vi "MAIN_Robot_Master.vi"() -> ()   [LabVIEW 2019]
uses:
  Type_defs/ESTADOS_ROBOT_MASTER.ctl
  Type_defs/TAREAS_ROBOT.ctl
  Type_defs/REFERENCIAS_CONTROLES_INDICADORES.ctl
  SHARED TYPES/Acciones_UI.ctl
  Type_defs/COMANDOS_TAREA.ctl
  <vilib>/Utility/error.llb/Error Cluster From Error Code.vi
  <vilib>/ErrorRing/Error Ring.xnode
  SHARED VI'S/SHARED VI'S.lvlib
  SHARED TYPES/SHARED TYPES.lvlib
panel:
  in  "Tab Control":enum32{"Page 1", "Page 2"}(tab)
  in  "Configurar estación":bool
  out "LABVIEW MESSAGES":string
  out "DISPOSITIVO CONECTADO":string
  out "ARDUINO MESSAGES":string
  in  "MOVIMIENTO MANUAL":bool
  in  "MOVER ASICS":bool
  in  "LEER QR":bool
  in  "TEST ASICS":bool
  in  "INICIAR COM":bool
  in  "Exit":bool
  out "ESTADO ACTUAL FSM":T1
  # "SISTEMA DE POSICIONAMIENTO AUTOMÁTICO DE ASICS"
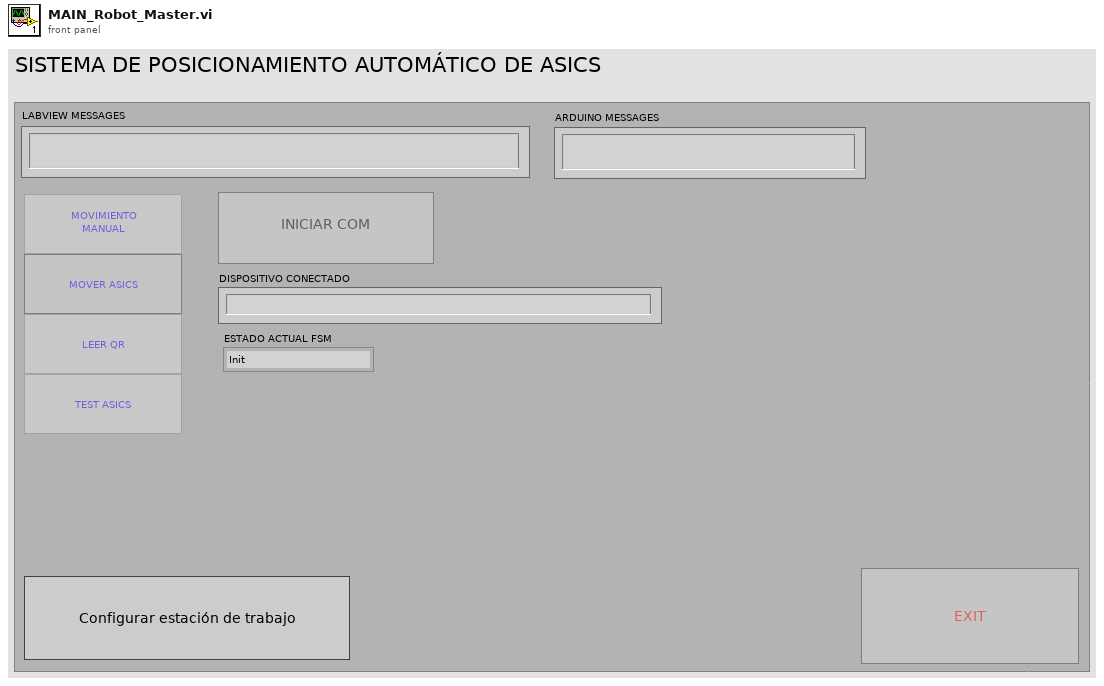
[diagram p1: front panel]
types:
  T1 = typedef "ESTADOS_ROBOT_MASTER.ctl" = enum16{"Init", "Iniciar Visa Arduino", "Sesiones Visa abiertas?", "Ping to Arduino", "Checkear config file", "Esperar_evento", "Tarea", "Exit", "Salir Arduino"}
  T2 = typedef "REFERENCIAS_CONTROLES_INDICADORES.ctl" = cluster{"LEER QR":refnum<vi>, "MOVER ASCIS":refnum<vi>, "CALIBRACION":refnum<vi>, "TEST ASICS":refnum<vi>, "EXIT":refnum<vi>, "AJUSTE CAM":refnum<vi>, "INICIAR COM":refnum<vi>, "ARDUINO MESSAGES":refnum<vi>, "LABVIEW MESSAGES":refnum<vi>, "DISPOSITIVO CONECTADO":refnum<vi>, "Config Estación":refnum<vi>}
  T3 = typedef "TAREAS_ROBOT.ctl" = enum16{"NINGUNA", "TEST ASICS", "AJUSTE CAM", "MOVER ASICS", "MOVIMIENTO MANUAL", "LEER QR", "CONFIG ESTACION"}
  T4 = typedef "SHARED TYPES.lvlib/Acciones_UI.ctl" = enum16{"Activar", "Desactivar", "Reiniciar default"}
  T5 = typedef "COMANDOS_TAREA.ctl" = enum16{"M", "T", "Q", "U", "S"}
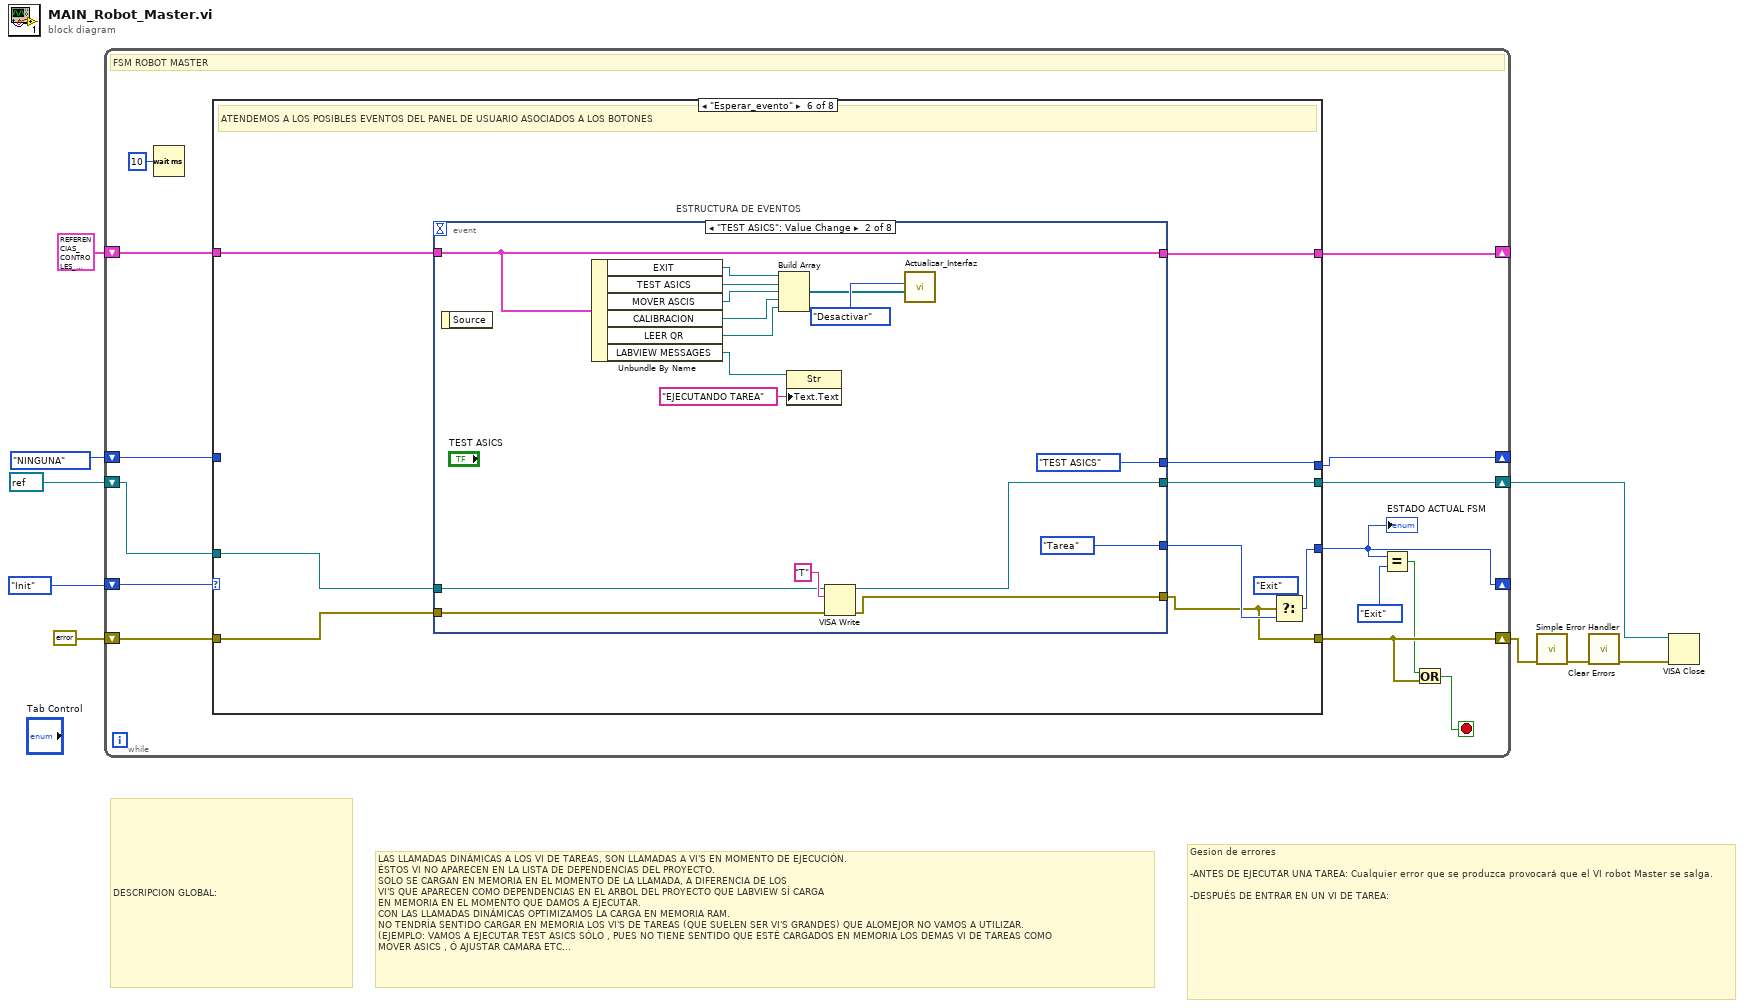
[diagram p0: block diagram]
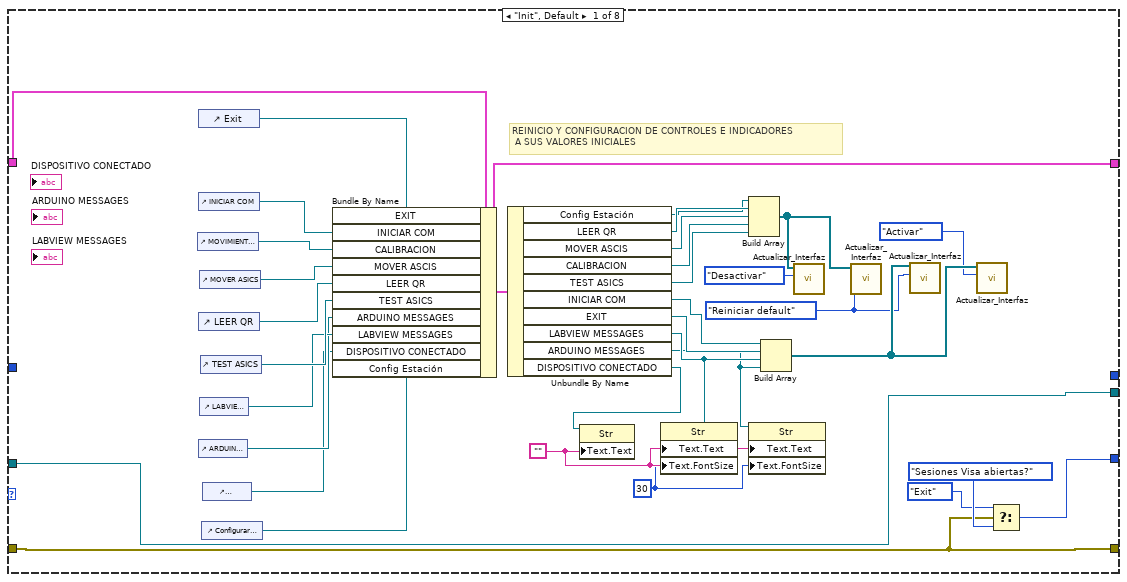
[diagram p2: hidden frame]
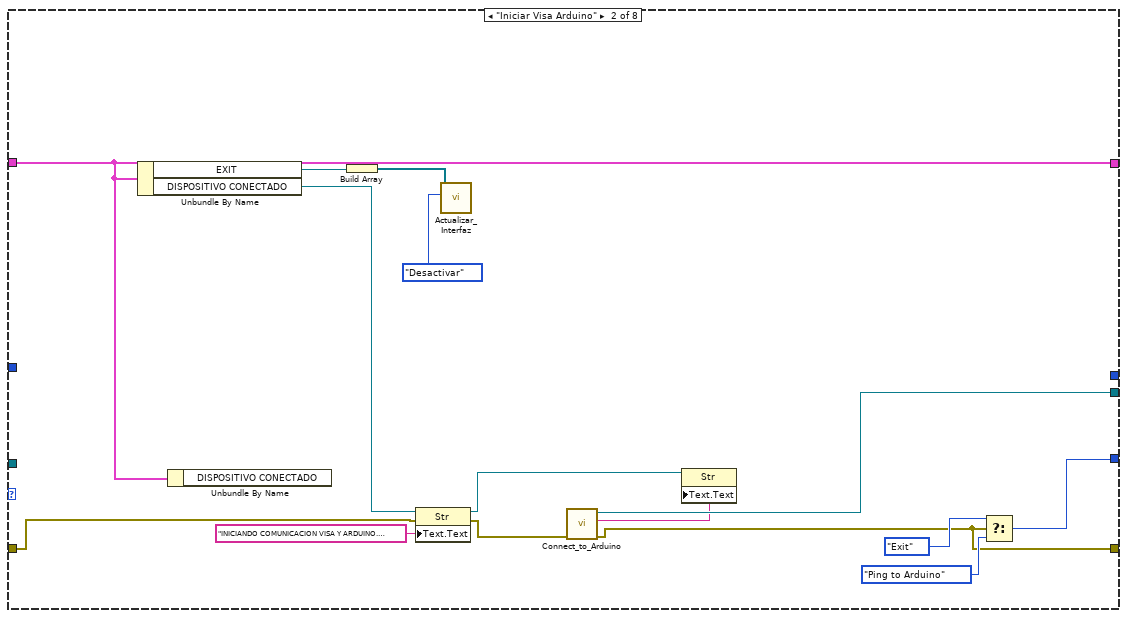
[diagram p3: hidden frame]
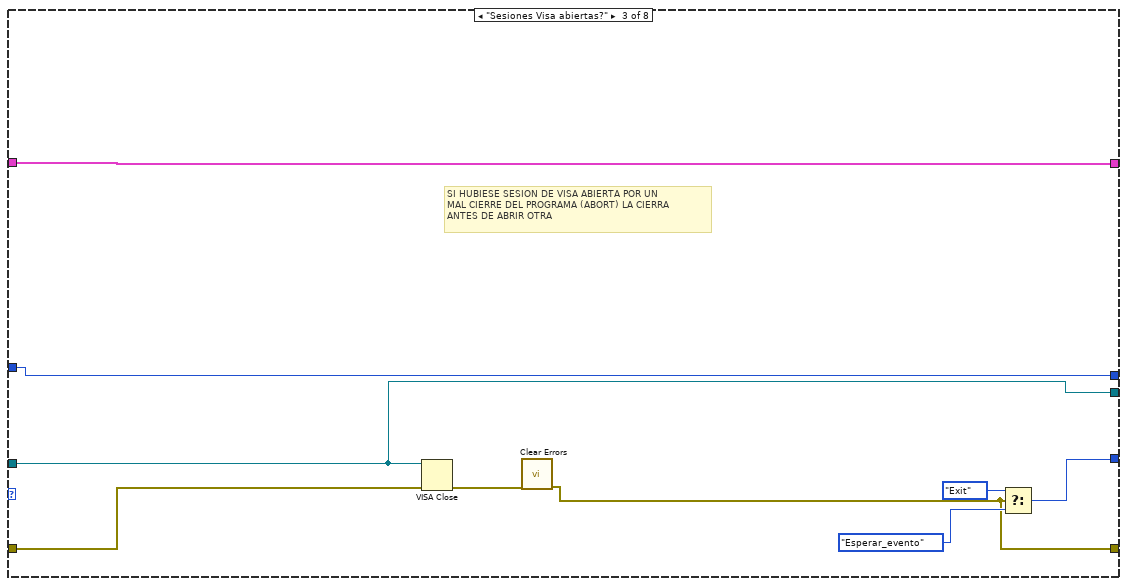
[diagram p4: hidden frame]
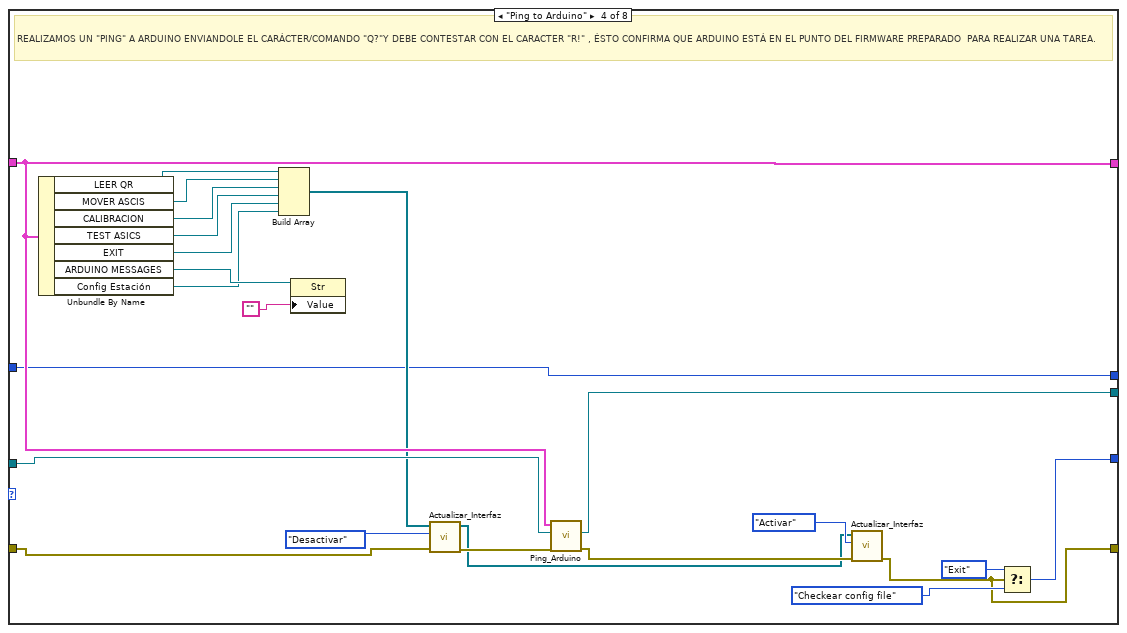
[diagram p5: hidden frame]
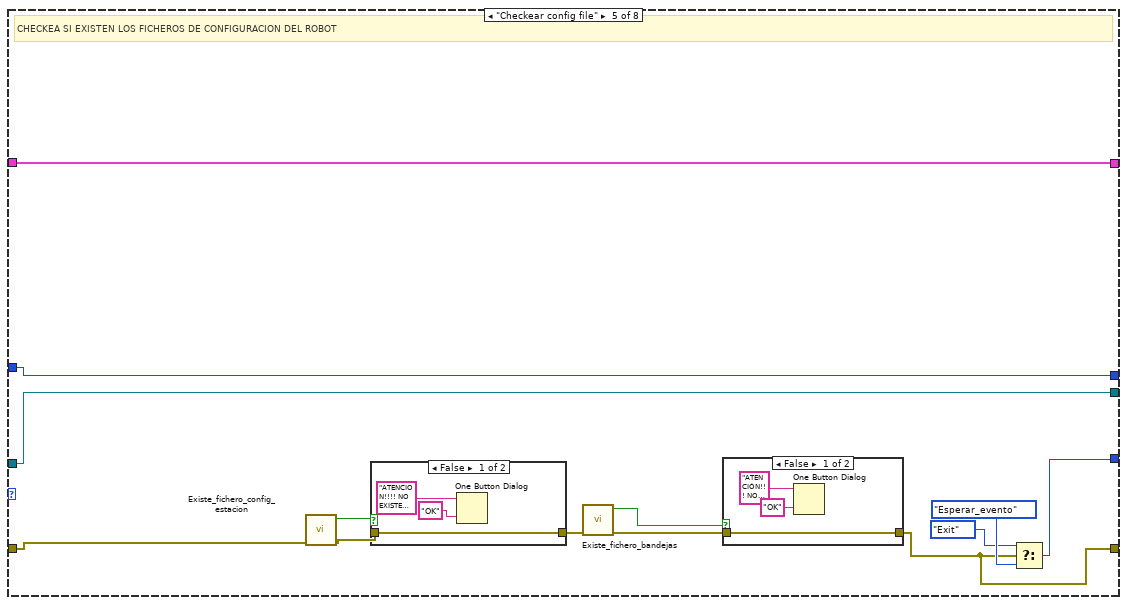
[diagram p6: hidden frame]
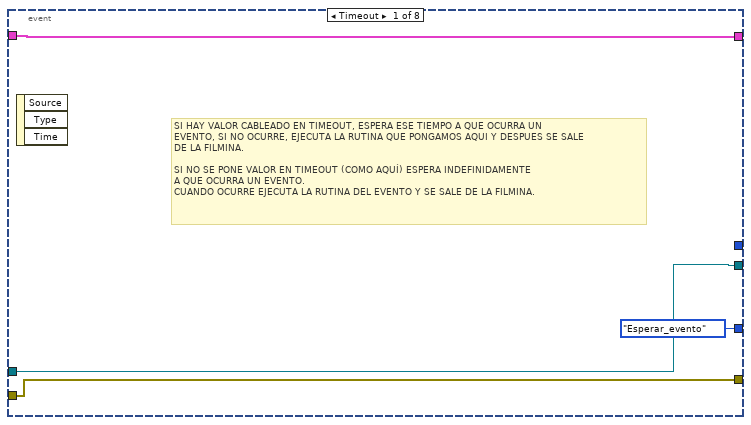
[diagram p9: hidden frame]
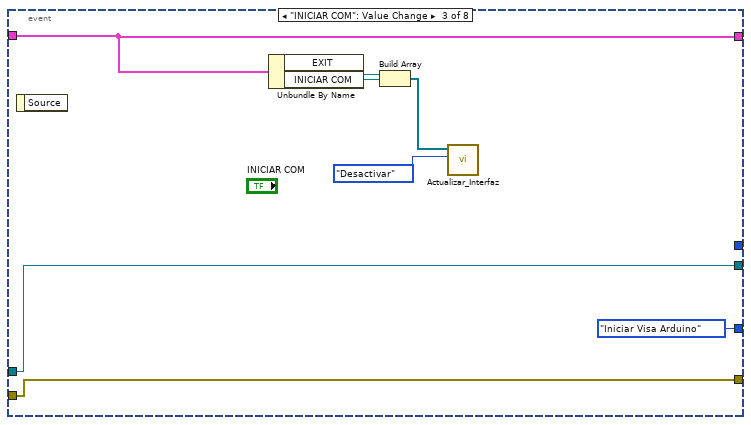
[diagram p10: hidden frame]
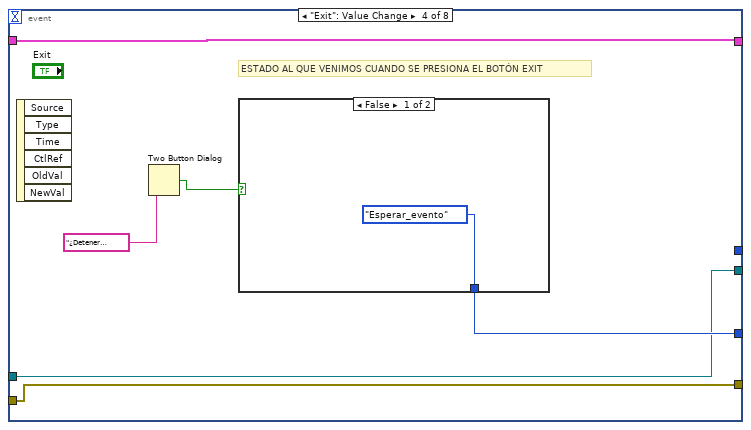
[diagram p11: hidden frame]
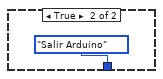
[diagram p12: hidden frame]
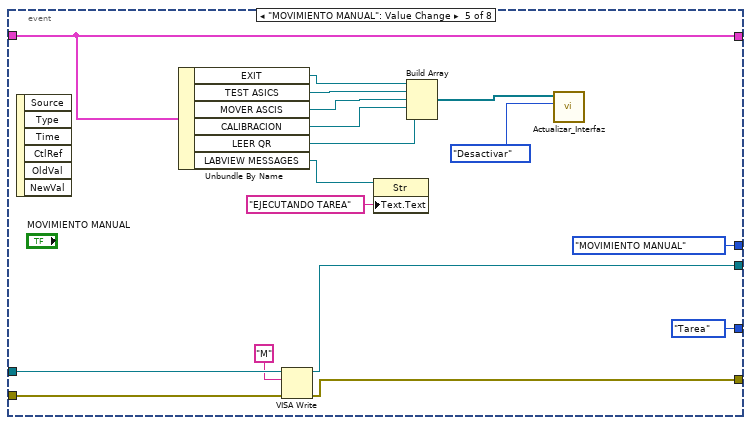
[diagram p13: hidden frame]
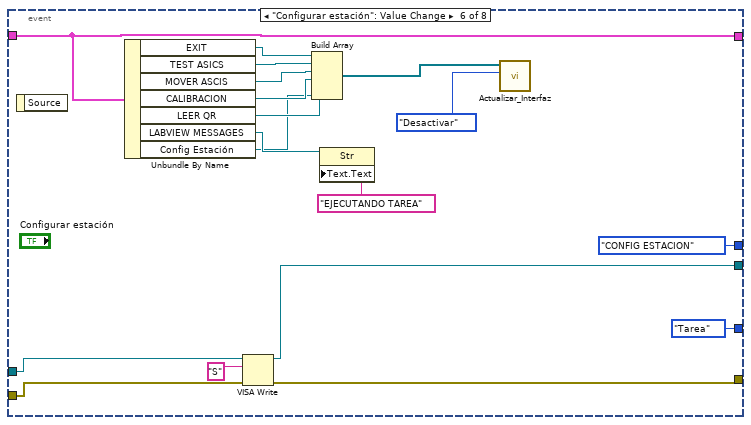
[diagram p14: hidden frame]
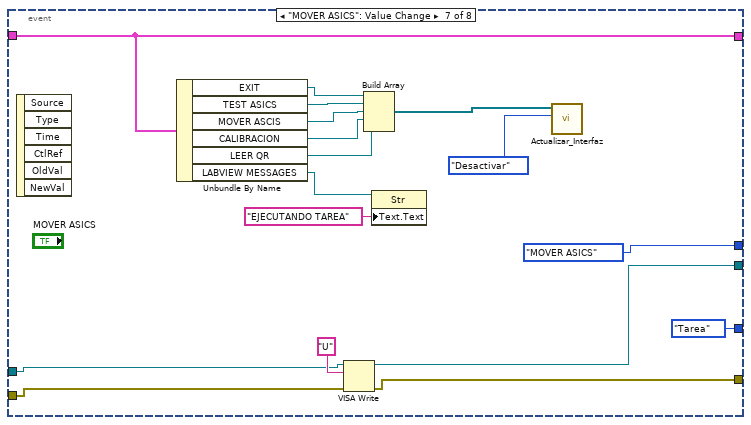
[diagram p15: hidden frame]
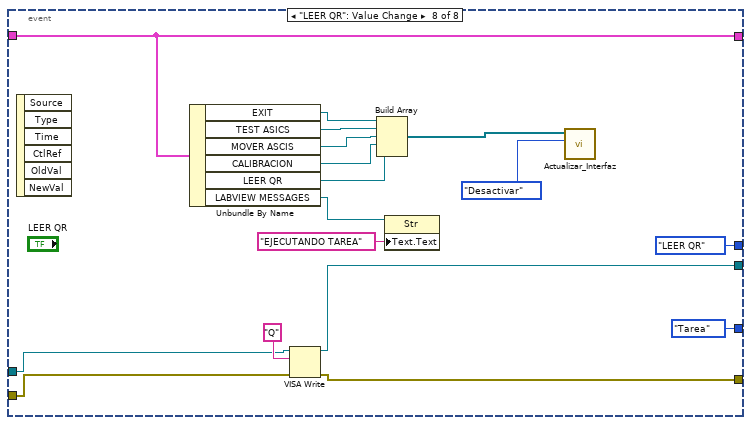
[diagram p16: hidden frame]
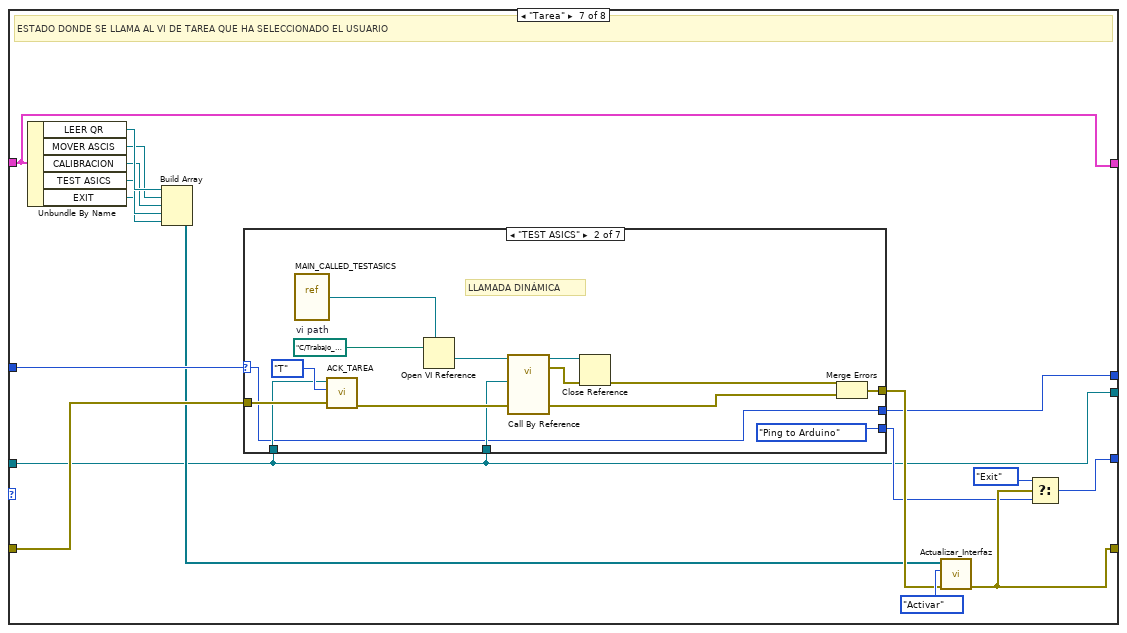
[diagram p17: hidden frame]
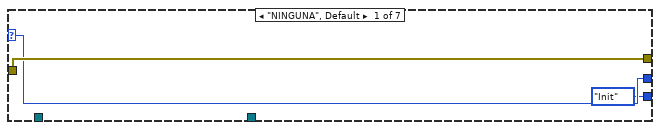
[diagram p18: hidden frame]
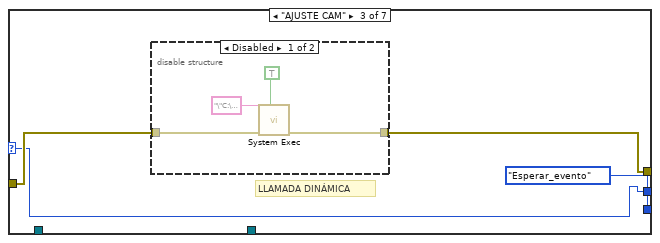
[diagram p19: hidden frame]
diagram:
  # "LAS LLAMADAS DINÁMICAS A LOS VI DE TAREAS, SON LLAMADAS A VI'S EN MOMENTO DE EJECUCIÓN.\nÉSTOS VI NO APARECEN EN LA LISTA DE DEPENDENCIAS DEL PROYECTO. \nSOLO SE CARGAN EN MEMORIA EN EL MOMENTO DE LA LLAMADA, A DIFERENCIA DE LOS\nVI'S QUE APARECEN COMO DEPENDENCIAS EN EL ARBOL DEL PROYECTO QUE LABVIEW SÍ CARGA\nEN MEMORIA EN EL MOMENTO QUE DAMOS A EJECUTAR.\nCON LAS LLAMADAS DINÁMICAS OPTIMIZAMOS LA CARGA EN MEMORIA RAM.\nNO TENDRÍA SENTIDO CARGAR EN MEMORIA LOS VI'S DE TAREAS (QUE SUELEN SER VI'S GRANDES) QUE ALOMEJOR NO VAMOS A UTILIZAR.\n(EJEMPLO: VAMOS A EJECUTAR TEST ASICS SÓLO , PUES NO TIENE SENTIDO QUE ESTÉ CARGADOS EN MEMORIA LOS DEMAS VI DE TAREAS COMO\nMOVER ASICS , Ó AJUSTAR CAMARA ETC..."
  # "Gesion de errores\n\n-ANTES DE EJECUTAR UNA TAREA: Cualquier error que se produzca provocará que el VI robot Master se salga.\n\n-DESPUÉS DE ENTRAR EN UN VI DE TAREA:"
  # "DESCRIPCION GLOBAL:"
  n1 = while {
    shift-right: [w15] -> _
    shift-left: ESTADOS_ROBOT_MASTER."Init" -> [w23]
    shift-right: [w18] -> w3
    shift-left: errorcluster {"status"=FALSE, "code"=0, "source"=""} ("error in (no error)") -> [w19]
    shift-right: [w20] -> _
    shift-left: T2 {"LEER QR"=refnum, "MOVER ASCIS"=refnum, "CALIBRACION"=refnum, "TEST ASICS"=refnum, "EXIT"=refnum, "AJUSTE CAM"=refnum, "INICIAR COM"=refnum, "ARDUINO MESSAGES"=refnum, "LABVIEW MESSAGES"=refnum, "DISPOSITIVO CONECTADO"=refnum, "Config Estación"=refnum} ("input cluster") -> [w21]
    shift-right: [w13] -> w2
    shift-left: refnum<visa-resource-name> refnum ("VISA resource name") -> [w10]
    shift-right: [w11] -> _
    shift-left: TAREAS_ROBOT."NINGUNA" -> [w12]
    stop <- w17 stop-if-true
    # "FSM ROBOT MASTER"
    n2 = Wait (ms)(milliseconds to wait=u32 10) -> ()  [unwired: 1 out]
    n3 = case shown="\"Esperar_evento\"" w23 {
      tunnel: w21 -> [w57 w67 w79 w102 w110 w135 w258 w359]
      tunnel: [w50 w67 w79 w102 w110 w134 w258 w359] -> w20
      tunnel: [w26 w58 w73 w85 w106 w127 w247 w355] -> w18
      tunnel: w19 -> [w26 w66 w81 w93 w117 w133 w245 w360]
      tunnel: [w27 w59 w74 w86 w105 w126 w248 ESTADOS_ROBOT_MASTER."Exit" ("Enum")] -> w15
      tunnel: w10 -> [w30 _ w78 w104 w109 w132 w243 w361]
      tunnel: [w30 w69 w78 w103 w109 w131 w243 w361] -> w13
      tunnel: w12 -> [_ _ w77 w89 w111 _ w250 w367]
      tunnel: [_ _ w77 w89 w111 w130 w242 w367] -> w11
      frame "Init", Default {
        w31 = 30
        w32 = ""
        w38 = Acciones_UI."Reiniciar default" ("Enum")
        # "REINICIO Y CONFIGURACION DE CONTROLES E INDICADORES\n A SUS VALORES INICIALES"
        n4 = control-ref of="MOVIMIENTO MANUAL"() -> (w54:refnum<vi>)
        n5 = control-ref of="Exit"() -> (w56:refnum<vi>)
        n6 = control-ref of="INICIAR COM"() -> (w55:refnum<vi>)
        n7 = control-ref of="LEER QR"() -> (w52:refnum<vi>)
        n8 = control-ref of="ARDUINO MESSAGES"() -> (w48:refnum<vi>)
        n9 = control-ref of="MOVER ASICS"() -> (w53:refnum<vi>)
        n10 = control-ref of="LABVIEW MESSAGES"() -> (w49:refnum<vi>)
        n11 = control-ref of="TEST ASICS"() -> (w51:refnum<vi>)
        n12 = control-ref of="Configurar estación"() -> (w25:refnum<vi>)
        n13 = control-ref of="DISPOSITIVO CONECTADO"() -> (w36:refnum<vi>)
        n14 = Bundle By Name(cluster=w57, "EXIT"=w56, "INICIAR COM"=w55, "CALIBRACION"=w54, "MOVER ASCIS"=w53, "LEER QR"=w52, "TEST ASICS"=w51, "ARDUINO MESSAGES"=w48, "LABVIEW MESSAGES"=w49, "DISPOSITIVO CONECTADO"=w36, "Config Estación"=w25) -> (w50:T2)
        n15 = Unbundle By Name(w50) -> ("Config Estación"=w24:refnum<vi>, "LEER QR"=w47:refnum<vi>, "MOVER ASCIS"=w46:refnum<vi>, "CALIBRACION"=w45:refnum<vi>, "TEST ASICS"=w44:refnum<vi>, "INICIAR COM"=w41:refnum<vi>, "EXIT"=w40:refnum<vi>, "LABVIEW MESSAGES"=w35:refnum<vi>, "ARDUINO MESSAGES"=w34:refnum<vi>, "DISPOSITIVO CONECTADO"=w33:refnum<vi>)
        n16 = property class="Str"(reference=w33, "Text.Text"=w32) -> ()  [unwired: 1 in, 2 out]
        n17 = property class="Str"(reference=w35, "Text.Text"=w32, "Text.FontSize"=w31) -> ()  [unwired: 1 in, 2 out]
        n18 = Build Array(w24, w47, w46, w45, w44) -> (w42:refnum<vi>[])
        n19 = property class="Str"(reference=w34, "Text.Text"=w32, "Text.FontSize"=w31) -> ()  [unwired: 1 in, 2 out]
        n20 = Build Array(w41, w40, w35, w34) -> (w39:refnum<vi>[])
        n21 = call "Actualizar_Interfaz.vi"("Enum"=Acciones_UI."Desactivar", "Controls"=w42) -> ()  [unwired: 8 in, 2 out]
        n22 = call "Actualizar_Interfaz.vi"("Enum"=w38, "Controls"=w42) -> ()  [unwired: 8 in, 2 out]
        n23 = call "Actualizar_Interfaz.vi"("Enum"=w38, "Controls"=w39) -> ()  [unwired: 8 in, 2 out]
        n24 = call "Actualizar_Interfaz.vi"("Enum"=Acciones_UI."Activar", "Controls"=w39) -> ()  [unwired: 8 in, 2 out]
        n25 = Select(t=ESTADOS_ROBOT_MASTER."Exit", s=w26, f=ESTADOS_ROBOT_MASTER."Sesiones Visa abiertas?" ("Enum")) -> (s? t:f=w27:T1)
      }
      frame "Iniciar Visa Arduino" {
        n26 = Unbundle By Name(w67) -> ("EXIT"=w72:refnum<vi>, "DISPOSITIVO CONECTADO"=w63:refnum<vi>)
        n27 = Unbundle By Name(w67) -> ()  [unwired: 1 out]
        n28 = Build Array(w72) -> (w71:refnum<vi>[])
        n29 = property class="Str"(reference=w63, error in=w66, "Text.Text"="INICIANDO COMUNICACION VISA Y ARDUINO. ESPERE...") -> (reference out=w62:refnum<vi>, error out=w64:errorcluster)
        n30 = call "Actualizar_Interfaz.vi"("Enum"=Acciones_UI."Desactivar", "Controls"=w71) -> ()  [unwired: 8 in, 2 out]
        n31 = call "Connect_to_Arduino.vi"("error in (no error)"=w64) -> ("error out"=w58:errorcluster, "DISPOSITIVO CONECTADO"=w68:string, "VISA Refnum out"=w69:refnum<visa-resource-name>)  [unwired: 8 in]
        n32 = property class="Str"(reference=w62, "Text.Text"=w68) -> ()  [unwired: 1 in, 2 out]
        n33 = Select(t=ESTADOS_ROBOT_MASTER."Exit", s=w58, f=ESTADOS_ROBOT_MASTER."Ping to Arduino" ("Enum")) -> (s? t:f=w59:T1)
      }
      frame "Sesiones Visa abiertas?" {
        # "SI HUBIESE SESION DE VISA ABIERTA POR UN \nMAL CIERRE DEL PROGRAMA (ABORT) LA CIERRA\nANTES DE ABRIR OTRA"
        n34 = VISA Close(VISA resource name=w78, error in (no error)=w81) -> (error out=w80:errorcluster)
        n35 = call <vilib>:"Clear Errors.vi"("error in (no error)"=w80) -> ("error out"=w73:errorcluster)  [unwired: 5 in, 1 out]
        n36 = Select(t=ESTADOS_ROBOT_MASTER."Exit", s=w73, f=ESTADOS_ROBOT_MASTER."Esperar_evento" ("Enum")) -> (s? t:f=w74:T1)
      }
      frame "Ping to Arduino" {
        # "REALIZAMOS UN \"PING\" A ARDUINO ENVIANDOLE EL CARÁCTER/COMANDO \"Q?\"Y DEBE CONTESTAR CON EL CARACTER \"R!\" , ÉSTO CONFIRMA QUE ARDUINO ESTÁ EN EL PUNTO DEL FIRMWARE PREPARADO  PARA REALIZAR UNA TAREA."
        n37 = Unbundle By Name(w102) -> ("LEER QR"=w101:refnum<vi>, "MOVER ASCIS"=w100:refnum<vi>, "CALIBRACION"=w99:refnum<vi>, "TEST ASICS"=w98:refnum<vi>, "EXIT"=w97:refnum<vi>, "ARDUINO MESSAGES"=w84:refnum<vi>, "Config Estación"=w82:refnum<vi>)
        n38 = Build Array(w101, w100, w99, w98, w97, w82) -> (w95:refnum<vi>[])
        n39 = property class="Str"(reference=w84, "Value"="") -> ()  [unwired: 1 in, 2 out]
        n40 = call "Actualizar_Interfaz.vi"("error in (no error)"=w93, "Enum"=Acciones_UI."Desactivar", "Controls"=w95) -> ("error out"=w94:errorcluster, "Controls 2"=w90:refnum<vi>[])  [unwired: 7 in]
        n41 = call "Ping_Arduino.vi"("error in (no error)"=w94, "VISA resource name"=w104, "input cluster"=w102) -> ("error IO"=w91:errorcluster, "VISA resource name out"=w103:refnum<visa-resource-name>)  [unwired: 7 in]
        n42 = call "Actualizar_Interfaz.vi"("error in (no error)"=w91, "Enum"=Acciones_UI."Activar", "Controls"=w90) -> ("error out"=w85:errorcluster)  [unwired: 7 in, 1 out]
        n43 = Select(t=ESTADOS_ROBOT_MASTER."Exit", s=w85, f=ESTADOS_ROBOT_MASTER."Checkear config file" ("Enum")) -> (s? t:f=w86:T1)
      }
      frame "Checkear config file" {
        # "CHECKEA SI EXISTEN LOS FICHEROS DE CONFIGURACION DEL ROBOT"
        n44 = call "Existe_fichero_config_estacion.vi"("Error In"=w117) -> ("Error Out"=w115:errorcluster, "file or folder exists?"=w116:bool)  [unwired: 9 in]
        n45 = case shown="False" w116 {
          tunnel: w115 -> [w122 w125]
          tunnel: [w122 w125] -> w114
          frame False {
            n46 = One Button Dialog(message="ATENCION!!!! NO EXISTE FICHERO DE CONFIGURACIÓN DE ESTACION\nEN EL DIRECTORIO RAÍZ DE ROBOT MASTER ", button name ("OK")="OK") -> ()  [unwired: 1 out]
          }
          frame True {
          }
        }
        n47 = call "Existe_fichero_bandejas.vi"("Error In"=w114) -> ("Error Out"=w112:errorcluster, "existe fichero bandejas?"=w113:bool)  [unwired: 9 in]
        n48 = case shown="False" w113 {
          tunnel: w112 -> [w118 w121]
          tunnel: [w118 w121] -> w106
          frame False {
            n49 = One Button Dialog(message="ATENCIÓN!!! NO EXISTE FICHERO DE CONFIGURACION DE BANDEJAS \".db\"\nEN EL DIRECTORIO RAIZ DE ROBOT MASTER.", button name ("OK")="OK") -> ()  [unwired: 1 out]
          }
          frame True {
          }
        }
        n50 = Select(t=ESTADOS_ROBOT_MASTER."Exit", s=w106, f=ESTADOS_ROBOT_MASTER."Esperar_evento" ("Enum")) -> (s? t:f=w105:T1)
      }
      frame "Esperar_evento" {
        # "ATENDEMOS A LOS POSIBLES EVENTOS DEL PANEL DE USUARIO ASOCIADOS A LOS BOTONES"
        n51 = event "ESTRUCTURA DE EVENTOS" shown="[1] \"TEST ASICS\": Value Change" {
          selector: _ -> [_ _ _ _ _ _ _ _]
          dyn-events: _ -> [_ _ _ _ _ _ _ _]
          timeout: _ -> [_ _ _ _ _ _ _ _]
          tunnel: w135 -> [w136 w147 w160 w165 w175 w192 w215 w232]
          tunnel: [ESTADOS_ROBOT_MASTER."Esperar_evento" ("Enum") ESTADOS_ROBOT_MASTER."Tarea" ("Enum") ESTADOS_ROBOT_MASTER."Iniciar Visa Arduino" ("Enum") w168 ESTADOS_ROBOT_MASTER."Tarea" ("Enum") ESTADOS_ROBOT_MASTER."Tarea" ("Enum") ESTADOS_ROBOT_MASTER."Tarea" ("Enum") ESTADOS_ROBOT_MASTER."Tarea" ("Enum")] -> w129
          tunnel: [w136 w147 w160 w165 w175 w192 w215 w232] -> w134
          tunnel: w133 -> [w139 w143 w157 w166 w178 w197 w212 w228]
          tunnel: [w139 w142 w157 w166 w176 w196 w209 w227] -> w127
          tunnel: w132 -> [w138 w141 w159 w167 w180 w198 w211 w226]
          tunnel: [w138 w140 w159 w167 w177 w195 w210 w225] -> w131
          tunnel: [_ TAREAS_ROBOT."TEST ASICS" _ _ TAREAS_ROBOT."MOVIMIENTO MANUAL" TAREAS_ROBOT."CONFIG ESTACION" TAREAS_ROBOT."MOVER ASICS" TAREAS_ROBOT."LEER QR"] -> w130
          event Timeout {
            # "SI HAY VALOR CABLEADO EN TIMEOUT, ESPERA ESE TIEMPO A QUE OCURRA UN \nEVENTO, SI NO OCURRE, EJECUTA LA RUTINA QUE PONGAMOS AQUI Y DESPUES SE SALE\nDE LA FILMINA.\n\nSI NO SE PONE VALOR EN TIMEOUT (COMO AQUÍ) ESPERA INDEFINIDAMENTE \nA QUE OCURRA UN EVENTO.\nCUANDO OCURRE EJECUTA LA RUTINA DEL EVENTO Y SE SALE DE LA FILMINA."
            n52 = event-data() -> ()  [unwired: 1 in, 3 out]
          }
          event "TEST ASICS": Value Change {
            n53 = event-data() -> ()  [unwired: 1 in, 1 out]
            n54 = Unbundle By Name(w147) -> ("EXIT"=w145:refnum<vi>, "TEST ASICS"=w154:refnum<vi>, "MOVER ASCIS"=w153:refnum<vi>, "CALIBRACION"=w152:refnum<vi>, "LEER QR"=w151:refnum<vi>, "LABVIEW MESSAGES"=w149:refnum<vi>)
            n55 = Build Array(w145, w154, w153, w152, w151) -> (w150:refnum<vi>[])
            n56 = property class="Str"(reference=w149, "Text.Text"="EJECUTANDO TAREA") -> ()  [unwired: 1 in, 2 out]
            n57 = VISA Write(VISA resource name=w141, write buffer="T", error in (no error)=w143) -> (VISA resource name out=w140:refnum<visa-resource-name>, error out=w142:errorcluster)  [unwired: 1 out]
            n58 = call "Actualizar_Interfaz.vi"("Enum"=Acciones_UI."Desactivar", "Controls"=w150) -> ()  [unwired: 8 in, 2 out]
          }
          event "INICIAR COM": Value Change {
            n59 = event-data() -> ()  [unwired: 1 in, 1 out]
            n60 = Unbundle By Name(w160) -> ("EXIT"=w163:refnum<vi>, "INICIAR COM"=w158:refnum<vi>)
            n61 = Build Array(w163, w158) -> (w162:refnum<vi>[])
            n62 = call "Actualizar_Interfaz.vi"("Enum"=Acciones_UI."Desactivar", "Controls"=w162) -> ()  [unwired: 8 in, 2 out]
          }
          event "Exit": Value Change {
            # "ESTADO AL QUE VENIMOS CUANDO SE PRESIONA EL BOTÓN EXIT"
            n63 = event-data() -> ()  [unwired: 1 in, 6 out]
            n64 = Two Button Dialog(message="¿Detener ejecución?") -> (T button?=w169:bool)  [unwired: 2 in]
            n65 = case shown="False" w169 {
              tunnel: [ESTADOS_ROBOT_MASTER."Esperar_evento" ("Enum") ESTADOS_ROBOT_MASTER."Salir Arduino" ("Enum")] -> w168
              frame False {
              }
              frame True {
              }
            }
          }
          event "MOVIMIENTO MANUAL": Value Change {
            n66 = event-data() -> ()  [unwired: 1 in, 6 out]
            n67 = Unbundle By Name(w175) -> ("EXIT"=w173:refnum<vi>, "TEST ASICS"=w188:refnum<vi>, "MOVER ASCIS"=w187:refnum<vi>, "CALIBRACION"=w186:refnum<vi>, "LEER QR"=w185:refnum<vi>, "LABVIEW MESSAGES"=w183:refnum<vi>)
            n68 = VISA Write(VISA resource name=w180, write buffer="M", error in (no error)=w178) -> (VISA resource name out=w177:refnum<visa-resource-name>, error out=w176:errorcluster)  [unwired: 1 out]
            n69 = property class="Str"(reference=w183, "Text.Text"="EJECUTANDO TAREA") -> ()  [unwired: 1 in, 2 out]
            n70 = Build Array(w173, w188, w187, w186, w185) -> (w184:refnum<vi>[])
            n71 = call "Actualizar_Interfaz.vi"("Enum"=Acciones_UI."Desactivar", "Controls"=w184) -> ()  [unwired: 8 in, 2 out]
          }
          event "Configurar estación": Value Change {
            n72 = event-data() -> ()  [unwired: 1 in, 1 out]
            n73 = Unbundle By Name(w192) -> ("EXIT"=w190:refnum<vi>, "TEST ASICS"=w206:refnum<vi>, "MOVER ASCIS"=w205:refnum<vi>, "CALIBRACION"=w204:refnum<vi>, "LEER QR"=w203:refnum<vi>, "LABVIEW MESSAGES"=w201:refnum<vi>, "Config Estación"=w191:refnum<vi>)
            n74 = VISA Write(VISA resource name=w198, write buffer="S", error in (no error)=w197) -> (VISA resource name out=w195:refnum<visa-resource-name>, error out=w196:errorcluster)  [unwired: 1 out]
            n75 = Build Array(w190, w206, w205, w204, w203, w191) -> (w202:refnum<vi>[])
            n76 = property class="Str"(reference=w201, "Text.Text"="EJECUTANDO TAREA") -> ()  [unwired: 1 in, 2 out]
            n77 = call "Actualizar_Interfaz.vi"("Enum"=Acciones_UI."Desactivar", "Controls"=w202) -> ()  [unwired: 8 in, 2 out]
          }
          event "MOVER ASICS": Value Change {
            n78 = event-data() -> ()  [unwired: 1 in, 6 out]
            n79 = Unbundle By Name(w215) -> ("EXIT"=w208:refnum<vi>, "TEST ASICS"=w223:refnum<vi>, "MOVER ASCIS"=w222:refnum<vi>, "CALIBRACION"=w221:refnum<vi>, "LEER QR"=w220:refnum<vi>, "LABVIEW MESSAGES"=w218:refnum<vi>)
            n80 = VISA Write(VISA resource name=w211, write buffer="U", error in (no error)=w212) -> (VISA resource name out=w210:refnum<visa-resource-name>, error out=w209:errorcluster)  [unwired: 1 out]
            n81 = Build Array(w208, w223, w222, w221, w220) -> (w219:refnum<vi>[])
            n82 = property class="Str"(reference=w218, "Text.Text"="EJECUTANDO TAREA") -> ()  [unwired: 1 in, 2 out]
            n83 = call "Actualizar_Interfaz.vi"("Enum"=Acciones_UI."Desactivar", "Controls"=w219) -> ()  [unwired: 8 in, 2 out]
          }
          event "LEER QR": Value Change {
            n84 = event-data() -> ()  [unwired: 1 in, 6 out]
            n85 = Unbundle By Name(w232) -> ("EXIT"=w230:refnum<vi>, "TEST ASICS"=w240:refnum<vi>, "MOVER ASCIS"=w239:refnum<vi>, "CALIBRACION"=w238:refnum<vi>, "LEER QR"=w237:refnum<vi>, "LABVIEW MESSAGES"=w235:refnum<vi>)
            n86 = VISA Write(VISA resource name=w226, write buffer="Q", error in (no error)=w228) -> (VISA resource name out=w225:refnum<visa-resource-name>, error out=w227:errorcluster)  [unwired: 1 out]
            n87 = Build Array(w230, w240, w239, w238, w237) -> (w236:refnum<vi>[])
            n88 = property class="Str"(reference=w235, "Text.Text"="EJECUTANDO TAREA") -> ()  [unwired: 1 in, 2 out]
            n89 = call "Actualizar_Interfaz.vi"("Enum"=Acciones_UI."Desactivar", "Controls"=w236) -> ()  [unwired: 8 in, 2 out]
          }
        }
        n90 = Select(t=ESTADOS_ROBOT_MASTER."Exit", s=w127, f=w129) -> (s? t:f=w126:T1)
      }
      frame "Tarea" {
        # "ESTADO DONDE SE LLAMA AL VI DE TAREA QUE HA SELECCIONADO EL USUARIO"
        n91 = Unbundle By Name(w258) -> ("LEER QR"=w257:refnum<vi>, "MOVER ASCIS"=w256:refnum<vi>, "CALIBRACION"=w255:refnum<vi>, "TEST ASICS"=w254:refnum<vi>, "EXIT"=w253:refnum<vi>)
        n92 = Build Array(w257, w256, w255, w254, w253) -> (w244:refnum<vi>[])
        n93 = case shown="\"TEST ASICS\"" w250 {
          selector: w250 -> [w260 w262 w277 w286 w301 w321 w336]
          tunnel: w245 -> [w261 w272 w278 w299 w309 w328 w353]
          tunnel: [w261 w275 w279 w290 w313 w334 w339] -> w251
          tunnel: w243 -> [_ w271 _ w289 w302 w327 w338]
          tunnel: [ESTADOS_ROBOT_MASTER."Init" ("Enum") ESTADOS_ROBOT_MASTER."Ping to Arduino" ("Enum") ESTADOS_ROBOT_MASTER."Esperar_evento" ("Enum") ESTADOS_ROBOT_MASTER."Ping to Arduino" ("Enum") ESTADOS_ROBOT_MASTER."Ping to Arduino" ("Enum") ESTADOS_ROBOT_MASTER."Ping to Arduino" ("Enum") ESTADOS_ROBOT_MASTER."Ping to Arduino" ("Enum")] -> w246
          tunnel: w243 -> [_ w263 _ w285 _ _ _]
          tunnel: [w260 w262 w277 w286 w301 w321 w336] -> w242
          frame "NINGUNA", Default {
          }
          frame "TEST ASICS" {
            w268 = path "C:/Trabajo_Robot/TFG_ROBOT/CONTROL_ROBOT/LVPROJ_TESTASICS/LABVIEW/MAIN_CALLED_TESTASICS.vi"  # vi path
            # "LLAMADA DINÁMICA"
            n94 = vi-ref "MAIN_CALLED_TESTASICS.vi"() -> (w267:refnum<vi>)
            n95 = call "ACK_TAREA.vi"("error in (no error)"=w272, "Enum"=COMANDOS_TAREA."T", "VISA resource name"=w271) -> ("error out"=w265:errorcluster)  [unwired: 7 in, 1 out]
            n96 = Open VI Reference(type specifier VI Refnum (for type only)=w267, vi path=w268) -> (vi reference=w266:refnum<vi>)  [unwired: 4 in, 1 out]
            n97 = call-by-ref "Call By Reference"(reference=w266, "Error In"=w265, "VISA resource name out"=w263) -> (reference out=w270:refnum<vi>, error out=w269:errorcluster, "Error Out"=w264:errorcluster)  [unwired: 10 in]
            n98 = Close Reference(reference=w270, error in (no error)=w269) -> (error out=w276:errorcluster)
            n99 = Merge Errors(w276, w264) -> (w275:errorcluster)
          }
          frame "AJUSTE CAM" {
            # "LLAMADA DINÁMICA"
            n100 = disable-structure shown="Disabled" {
              disable-tunnel: [w284 _] -> w279
              disable-tunnel: w278 -> [w283 _]
              frame Disabled {
                n101 = call <vilib>:"System Exec.vi"("wait until completion? (T)"=TRUE, "error in (no error)"=w283, "command line"="\"C:\\Program Files\\Notepad++\\notepad++.exe\"DinoCapture.exe") -> ("error out"=w284:errorcluster)  [unwired: 5 in, 3 out]
              }
              frame Enabled {
              }
            }
          }
          frame "MOVER ASICS" {
            # "LLAMADA DINÁMICA"
            n102 = call "ACK_TAREA.vi"("error in (no error)"=w299, "Enum"=COMANDOS_TAREA."U", "VISA resource name"=w289) -> ("error out"=w297:errorcluster)  [unwired: 7 in, 1 out]
            n103 = vi-ref "MAIN_CALLED.vi"() -> (w298:refnum<vi>)
            n104 = Open VI Reference(type specifier VI Refnum (for type only)=w298, vi path=path "C:/Trabajo_Robot/TFG_ROBOT/CONTROL_ROBOT/LVPROJ_TRASPASO_ASICS/LABVIEW_STANDALONE/MAIN_CALLED.vi", error in (no error)=w297) -> (vi reference=w296:refnum<vi>, error out=w295:errorcluster)  [unwired: 3 in]
            n105 = call-by-ref "?"(reference=w296, "Error In"=w295, "SESION VISA"=w285) -> (reference out=w294:refnum<vi>, error out=w293:errorcluster, "Error Out"=w291:errorcluster)  [unwired: 10 in]
            n106 = Close Reference(reference=w294, error in (no error)=w293) -> (error out=w292:errorcluster)
            n107 = Merge Errors(w292, w291) -> (w290:errorcluster)
          }
          frame "MOVIMIENTO MANUAL" {
            # "LLAMADA DINÁMICA"
            n108 = vi-ref "MAIN_call.vi"() -> (w306:refnum<vi>)
            n109 = call "ACK_TAREA.vi"("error in (no error)"=w309, "Enum"=COMANDOS_TAREA."M", "VISA resource name"=w302) -> ("error out"=w308:errorcluster)  [unwired: 7 in, 1 out]
            n110 = Open VI Reference(type specifier VI Refnum (for type only)=w306, vi path=path "C:/Trabajo_Robot/TFG_ROBOT/CONTROL_ROBOT/LVPROJ_MOVIMIENTO_CABEZAL/LABVIEW_MOVIMIENTO/MOVIMIENTO CABEZAL/MAIN_call.vi") -> (vi reference=w320:refnum<vi>, error out=w318:errorcluster)  [unwired: 4 in]
            n111 = invoke class="VI (strict)" method="FP.Open"(reference=w320, error in=w318, "Activate"=TRUE ("Activate?")) -> (reference out=w305:refnum<vi>, error out=w317:errorcluster)  [unwired: 2 in, 3 out]
            n112 = call-by-ref "?"(reference=w305, error in=w317, "error IO"=w308, "Modo"=w301, "VISA SESSION"=w302) -> (reference out=w316:refnum<vi>, error out=w315:errorcluster, 0:"error out"=w314:errorcluster)  [unwired: 7 in, 1 out]
            n113 = invoke class="VI (strict)" method="FP.Close"(reference=w316, error in=w315) -> (reference out=w311:refnum<vi>, error out=w312:errorcluster)  [unwired: 1 in, 1 out]
            n114 = Close Reference(reference=w311, error in (no error)=w312) -> (error out=w310:errorcluster)
            n115 = Merge Errors(w310, w314) -> (w313:errorcluster)
          }
          frame "LEER QR" {
            # "LLAMADA DINÁMICA"
            n116 = vi-ref "MAIN_CALLED_leerQR.vi"() -> (w324:refnum<vi>)
            n117 = call "ACK_TAREA.vi"("error in (no error)"=w328, "Enum"=COMANDOS_TAREA."Q", "VISA resource name"=w327) -> ("error out"=w326:errorcluster)  [unwired: 7 in, 1 out]
            n118 = Open VI Reference(type specifier VI Refnum (for type only)=w324, vi path=path "C:/Trabajo_Robot/TFG_ROBOT/CONTROL_ROBOT/LVPROJ_LEER_QR/LABVIEW/MAIN_CALLED_leerQR.vi", error in (no error)=w326) -> (vi reference=w322:refnum<vi>, error out=w323:errorcluster)  [unwired: 3 in]
            n119 = call-by-ref "?"(reference=w322, "Error In"=w323, "VISA resource name out"=w327) -> (reference out=w332:refnum<vi>, error out=w331:errorcluster, "Error Out"=w330:errorcluster)  [unwired: 10 in]
            n120 = Close Reference(reference=w332, error in (no error)=w331) -> (error out=w335:errorcluster)
            n121 = Merge Errors(w335, w330) -> (w334:errorcluster)
          }
          frame "CONFIG ESTACION" {
            n122 = vi-ref "Main.vi"() -> (w352:refnum<vi>)
            n123 = call "ACK_TAREA.vi"("error in (no error)"=w353, "Enum"=COMANDOS_TAREA."S", "VISA resource name"=w338) -> ("error out"=w342:errorcluster)  [unwired: 7 in, 1 out]
            n124 = Open VI Reference(type specifier VI Refnum (for type only)=w352, vi path=path "C:/Trabajo_Robot/TFG_ROBOT/CONTROL_ROBOT/LVPROJ_CONFIG_ESTACION/Main.vi") -> (vi reference=w350:refnum<vi>, error out=w346:errorcluster)  [unwired: 4 in]
            n125 = invoke class="VI (strict)" method="FP.Open"(reference=w350, error in=w346) -> (reference out=w349:refnum<vi>, error out=w345:errorcluster)  [unwired: 3 in, 3 out]
            n126 = call-by-ref "?"(reference=w349, error in=w345, 8:"error in (no error)"=w342, "MODO"=w336, "VISA sesion"=w338) -> (reference out=w348:refnum<vi>, error out=w344:errorcluster, 0:"error out"=w341:errorcluster)  [unwired: 7 in, 1 out]
            n127 = invoke class="VI (strict)" method="FP.Close"(reference=w348, error in=w344) -> (reference out=w347:refnum<vi>, error out=w343:errorcluster)  [unwired: 1 in, 1 out]
            n128 = Close Reference(reference=w347, error in (no error)=w343) -> (error out=w340:errorcluster)
            n129 = Merge Errors(w340, w341) -> (w339:errorcluster)
          }
        }
        n130 = call "Actualizar_Interfaz.vi"("error in (no error)"=w251, "Enum"=Acciones_UI."Activar", "Controls"=w244) -> ("error out"=w247:errorcluster)  [unwired: 7 in, 1 out]
        n131 = Select(t=ESTADOS_ROBOT_MASTER."Exit", s=w247, f=w246) -> (s? t:f=w248:T1)
      }
      frame "Salir Arduino" {
        w364 = "E" ("write buffer")
        n132 = VISA Clear(VISA resource name=w361, error in (no error)=w360) -> (error out=w362:errorcluster)  [unwired: 1 out]
        n133 = VISA Write(VISA resource name=w361, write buffer=w364, error in (no error)=w362) -> (return count=w366:u32, error out=w363:errorcluster)  [unwired: 1 out]
        n134 = VISA Read(VISA resource name=w361, byte count=w366, error in (no error)=w363) -> (read buffer=w365:string, error out=w356:errorcluster)  [unwired: 2 out]
        n135 = Equal?(x=w365, y=w364) -> (x = y?=w358:bool)
        n136 = case shown="False" w358 {
          tunnel: [w369 _] -> w357
          frame False {
            n137 = xnode "Error Ring"() -> ("error out"=w369:errorcluster)
          }
          frame True {
            n138 = property on="ARDUINO MESSAGES" class="Str"("Value"="COMANDO EXIT RECIBIDO CORRECTAMENTE" ("MENSAJES AL USUARIO")) -> ()  [unwired: 2 in, 2 out]
            n139 = property on="LABVIEW MESSAGES" class="Str"("Value"="VI DETENIDO CORRECTAMENTE...SALIENDO" ("MENSAJES AL USUARIO")) -> ()  [unwired: 2 in, 2 out]
            n140 = call "Time Delay"() -> ()  [unwired: 11 in, 1 out]
          }
        }
        n141 = Merge Errors(w357, w356) -> (w355:errorcluster)
      }
    }
    "ESTADO ACTUAL FSM" <- w15
    n142 = Equal?(x=w15, y=ESTADOS_ROBOT_MASTER."Exit") -> (x = y?=w14:bool)
    n143 = Or(x=w14, y=w18) -> (x .or. y?=w17:bool)
  }
  n144 = call <vilib>:"Simple Error Handler.vi"("error in (no error)"=w3) -> ("error out"=w4:errorcluster)  [unwired: 4 in, 4 out]
  n145 = call <vilib>:"Clear Errors.vi"("error in (no error)"=w4) -> ("error out"=w5:errorcluster)  [unwired: 5 in, 1 out]
  n146 = VISA Close(VISA resource name=w2, error in (no error)=w5) -> ()  [unwired: 1 out]
